vi "yokogawa file save to usb.vi"() -> ()   [LabVIEW 2011]
panel:
  in  "Select Trace (0: Trace A)":u16(ring) items=["Trace D", "Trace B", "Trace C", "Trace D", "Trace E", "Trace F", "Trace G"]
  out "Error Out":errorcluster
  in  "File Name (USB has to be NTFS format)":string="20150311-#8-fiber-#1"
  in  "Error In":errorcluster
  in  "VISA session":refnum<visa-resource-name>="GPIB0::1::INSTR"
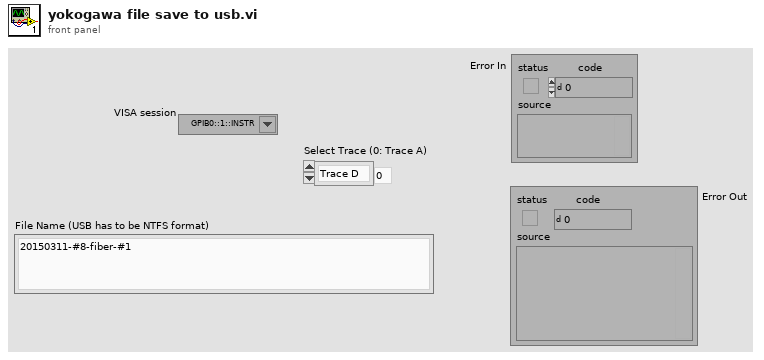
[diagram p1: front panel]
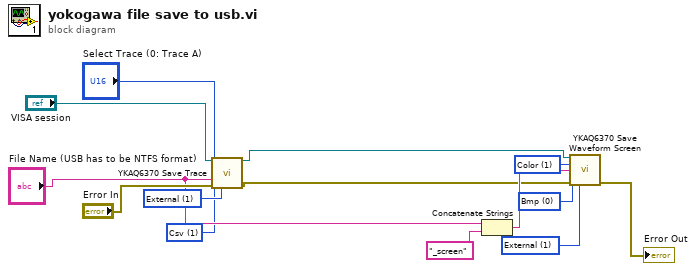
[diagram p0: block diagram]
diagram:
  w2 = u16 1 items=["Bin", "Csv"] ("File Type (0: Bin)")
  w3 = u16 1 items=["Internal", "External"] ("Current Drive (0: Internal)")
  w4 = u16 1 items=["Internal", "External"] ("Current Drive (0: Internal)")
  w8 = u16 0 items=["Bmp", "Tiff"] ("File Type (0: Bmp)")
  w9 = u16 1 items=["B&W", "Color"] ("Color Mode (1: Color)")
  n1 = call <instrlib>:"YKAQ6370 Save Trace.vi"("VISA resource name"="VISA session", "Select Trace (0: Trace A)"="Select Trace (0: Trace A)", "File Type (0: Bin)"=w2, "File Name (empty)"="File Name (USB has to be NTFS format)", "error in (no error)"="Error In", "Current Drive (0: Internal)"=w4) -> ("VISA resource name out"=w5:refnum<visa-resource-name>, "error out"=w6:errorcluster)  [unwired: 8 in]
  n2 = Concatenate Strings("File Name (USB has to be NTFS format)", "_screen" ("string")) -> (w10:string)
  n3 = call <instrlib>:"YKAQ6370 Save Waveform Screen.vi"("VISA resource name"=w5, "Color Mode (1: Color)"=w9, "File Name (empty)"=w10, "File Type (0: Bmp)"=w8, "error in (no error)"=w6, "Current Drive (0: Internal)"=w3) -> ("error out"=→"Error Out":errorcluster)  [unwired: 8 in, 1 out]
